vi "Create Python Graph (Example).vi"() -> ()   [LabVIEW 2013]
panel:
  out "Error OUT":errorcluster
  out "Command Line Error":string
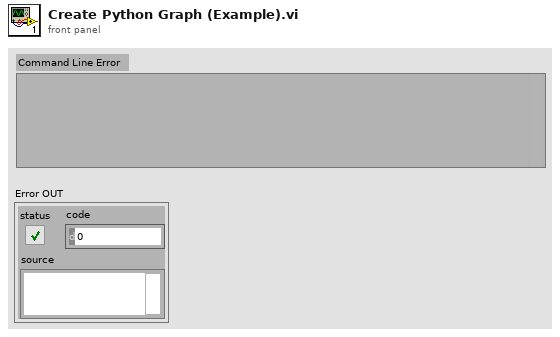
[diagram p1: front panel]
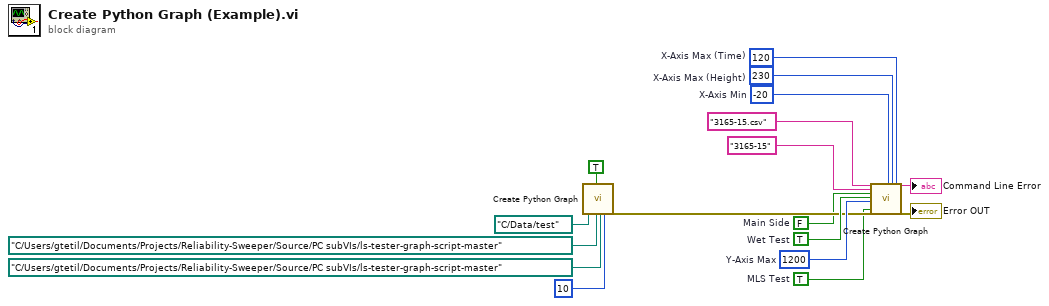
[diagram p0: block diagram]
diagram:
  w1 = 120  # X-Axis Max (Time)
  w2 = 230  # X-Axis Max (Height)
  w3 = -20  # X-Axis Min
  w7 = TRUE  # MLS Test
  w6 = FALSE  # Main Side
  w16 = 1200  # Y-Axis Max
  w17 = TRUE  # Wet Test
  n1 = call "Create Python Graph.vi"("Data Base Path"=path "C:/Data/test", "Init (F)"=TRUE, "Tolerances Path"=path "C:/Users/gtetil/Documents/Projects/Reliability-Sweeper/Source/PC subVIs/ls-tester-graph-script-master" ("Python Script Directory"), "Python Script Directory"=path "C:/Users/gtetil/Documents/Projects/Reliability-Sweeper/Source/PC subVIs/ls-tester-graph-script-master", "Data Start Index"=u32 10) -> ("Error OUT"=w9:errorcluster)  [unwired: 21 in, 1 out]
  n2 = call "Create Python Graph.vi"("File Name"="3165-15.csv", "Title"="3165-15" ("File Name"), "Main Side"=w6, "Wet Test"=w17, "Y-Axis Max"=w16, "MLS Test"=w7, "Error IN"=w9, "X-Axis Min"=w3, "X-Axis Max (Height)"=w2, "X-Axis Max (Time)"=w1) -> ("Command Line Error"=→"Command Line Error":string, "Error OUT"=→"Error OUT":errorcluster)  [unwired: 16 in]
